vi "Sync Lock.vi"(8 "error in (no error)":errorcluster, 9 "Timeout (-1ms)":i32=-1, 11 "Instrument Owner in":refnum<class "Instrument Owner.lvclass">) -> (0 "error out":errorcluster, 1 "Success?":bool, 3 "Instrument Owner out":refnum<class "Instrument Owner.lvclass">)   [LabVIEW 2020, in "Instrument Handler.lvlib" / "Instrument Owner.lvclass"]
doc: "Aquire the Enqueue Lock semaphore and clear the Enqueue Sync Notifier before enqueue on the Instrument Sequencer."
uses:
  Instrument Owner.lvclass
  Instrument Owner.lvclass/Instrument Owner.ctl
  PPL/HDH.Data.Generic.lvlibp/Synchronization/Notifier/Notifier.lvclass
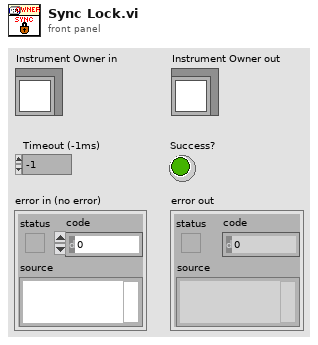
[diagram p1: front panel]
types:
  T1 = typedef "Instrument Handler.lvlib/Ctl_InstrumentSynchronicationCluster.ctl" = cluster{"Launched?":bool, "Driver Path":path, "Alias":string, "Connection Type":T2, "Pre Initialization Data":variant, "Enqueue Sync":refnum<class "Notifier.lvclass">, "Enqueue Lock":T3, "Owner Enqueuer":refnum<class "Message Enqueuer.lvclass">, "Owner":refnum<class "Sequencer Core.lvclass">, "Instrument ID":u32}
  T2 = typedef "HDH.Actor Framework.Core.Instrument Driver.lvlibp/Instrument Driver.lvclass/Ctl_ConnectionType.ctl" = enum16{"BuiltIn/System", "PXI/PCI", "USB", "GPIB", "VXI", "Serial", "TCP/IP", "cRIO", "SCXI", "cDAQ", "SwitchBlock", "SCC", "FireWire", "Accessory", "CAN", "SwitchBlock Device"}
  T3 = typedef "Semaphore RefNum" = refnum<k1>
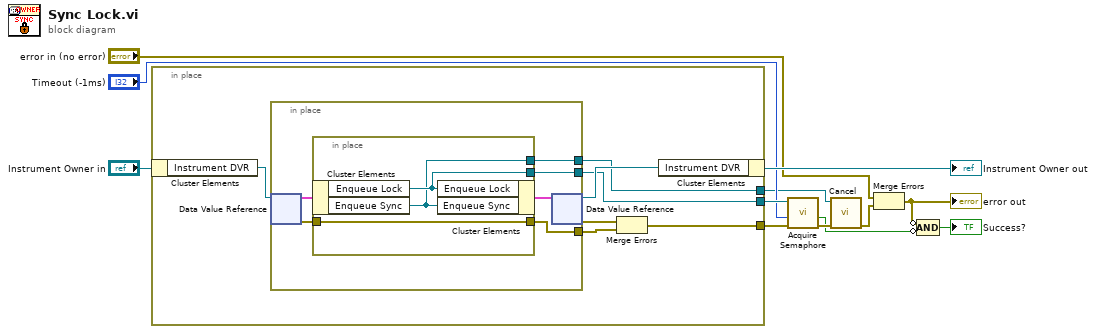
[diagram p0: block diagram]
diagram:
  n1 = in-place {
    in-place-border: [w16] -> w5
    in-place-border: [w14] -> w7
    in-place-border: [w13] -> w4
    n2 = in-place-cluster #1("Instrument Owner in") -> ("Instrument DVR"=w18:refnum<data-value>)
    n3 = in-place {
      in-place-border: [w25] -> w19
      in-place-border: [w21] -> w14
      in-place-border: [w20] -> w13
      n4 = in-place-dvr #2(w18) -> (w24:T1, w22:errorcluster)
      n5 = in-place {
        in-place-border: [w28] -> w25
        in-place-border: w22 -> [w28]
        in-place-border: [w27] -> w21
        in-place-border: [w26] -> w20
        n6 = in-place-cluster #3(w24) -> ("Enqueue Lock"=w27:T3, "Enqueue Sync"=w26:refnum<class "Notifier.lvclass">)
        n7 = in-place-cluster #3("Enqueue Lock"=w27, "Enqueue Sync"=w26) -> (w23:T1)
      }
      n8 = in-place-dvr #2(w23) -> (w17:refnum<data-value>, w15:errorcluster)
    }
    n9 = Merge Errors(w15, w19) -> (w16:errorcluster)
    n10 = in-place-cluster #1("Instrument DVR"=w17) -> (→"Instrument Owner out":refnum<class "Instrument Owner.lvclass">)
  }
  n11 = call <vilib>:"Acquire Semaphore.vi"("error in (no error)"=w5, "ms timeout (-1)"="Timeout (-1ms)", "semaphore"=w7) -> ("error out"=w3:errorcluster, "timed out"=w2:bool)  [unwired: 2 in, 1 out]
  n12 = call "Cancel.vi"("error in (no error)"=w3, "Notifier in"=w4) -> ("error out"=w1:errorcluster)  [unwired: 7 in, 2 out]
  n13 = Merge Errors("error in (no error)", w1) -> (w9:errorcluster)
  "error out" <- w9
  n14 = Compound Arithmetic op=AND(invert w9, invert w2) -> (→"Success?":bool)
